vi "Function Template.vi"(8 "Error In":errorcluster, 11 "Data In":T2) -> (0 "Error Out":errorcluster, 3 "Data Out":T2)   [LabVIEW 2019]
doc: "Description of VI"
uses:
  Controls/Data.ctl
  <vilib>/Utility/error.llb/DialogType.ctl
  <vilib>/Utility/miscctls.llb/LVPointTypeDef.ctl
panel:
  out "Control Tab":T1(tab)
  out "Console Out":string
  out "Error Message":string
  out "VI-filename":string
  out "Revision Number":u32
  out "VI Description":string
  out "Callers' Names":string[](array[string])
  out "Code Size":u32
  out "VI Type":T3(ring)
  out "Project name":string
  out "Project filepath":path
  out "VI filepath":path
  out "Project Description":string
  out "VI-Name":string
  # "Common Errors:"
  # "0:"
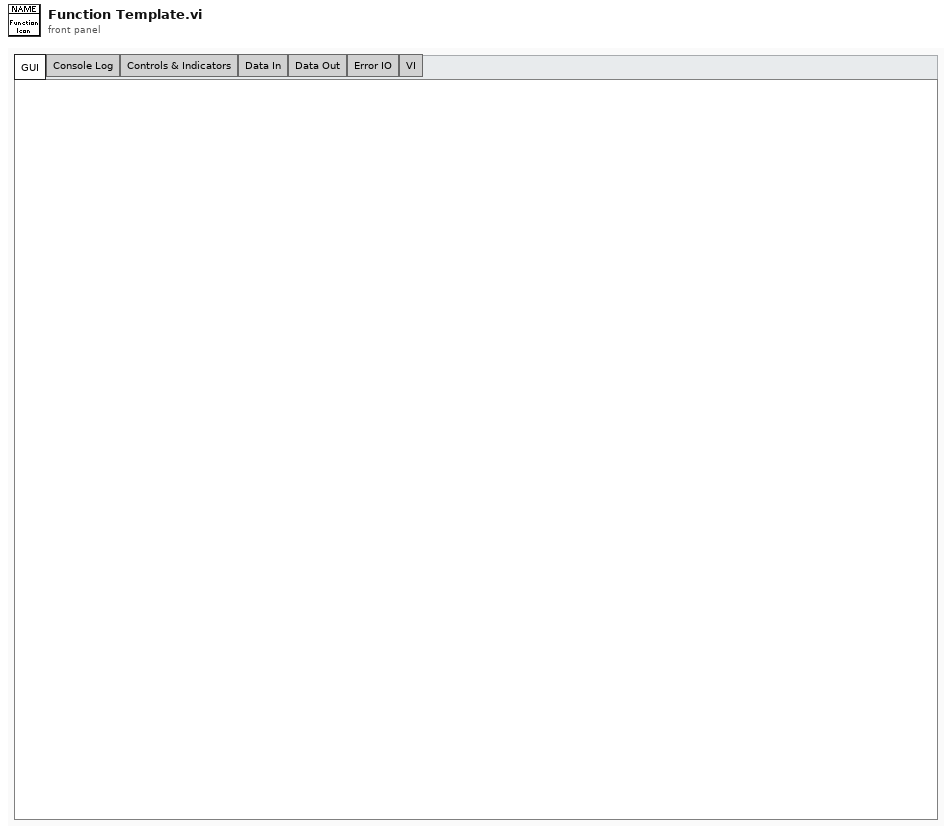
[diagram p1: front panel]
types:
  T1 = enum32{"GUI", "Console Log", "Controls & Indicators", "Data In", "Data Out", "Error IO", "VI"}
  T2 = typedef "Data.ctl" = cluster{"Console log":string}
  T3 = enum32{"invalid VI type", "Standard VI", "Control VI", "Global VI", "Polymorphic VI", "Configuration VI", "SubSystem", "Facade VI", "Method VI", "Statechart Diagram VI"}
  T4 = typedef "LVPointTypeDef.ctl" = cluster{"Horizontal":i16, "Vertical":i16}
  T5 = typedef "DialogType.ctl" = u16
  T6 = typedef "LVRectTypeDef.ctl" = cluster{"Left":i16, "Top":i16, "Right":i16, "Bottom":i16}
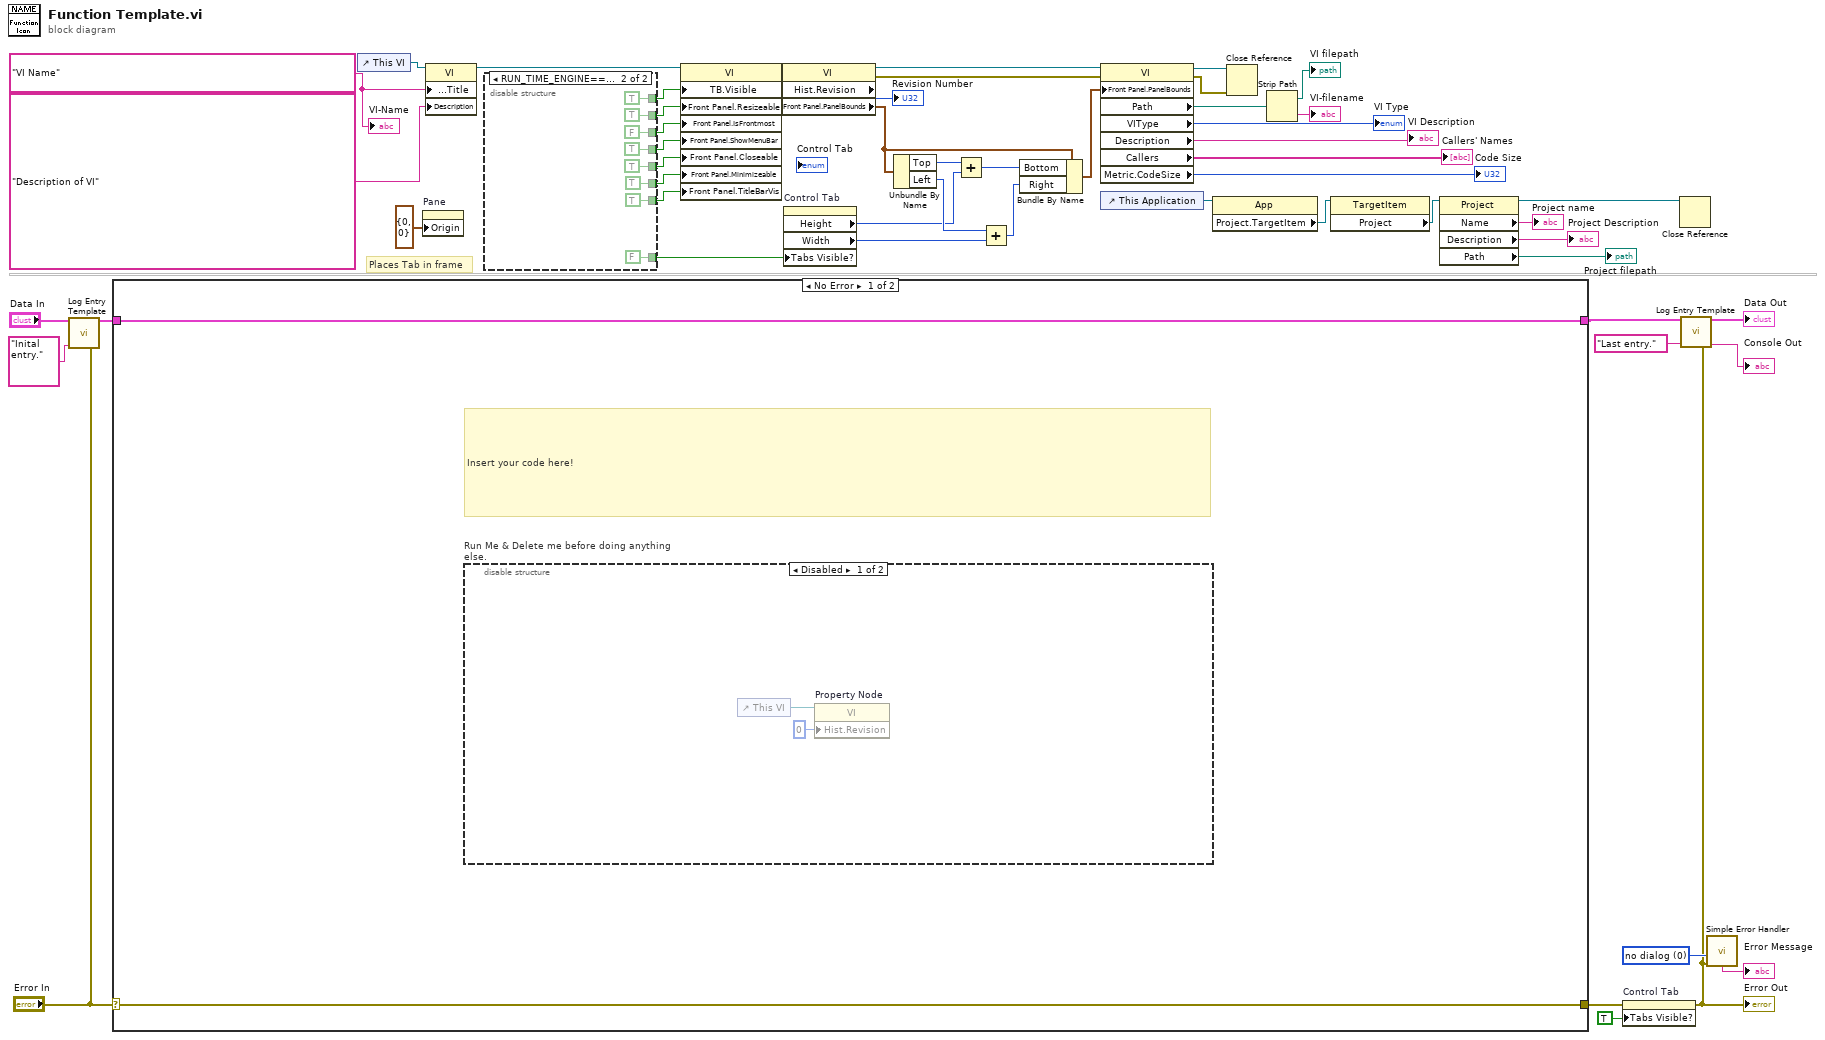
[diagram p0: block diagram]
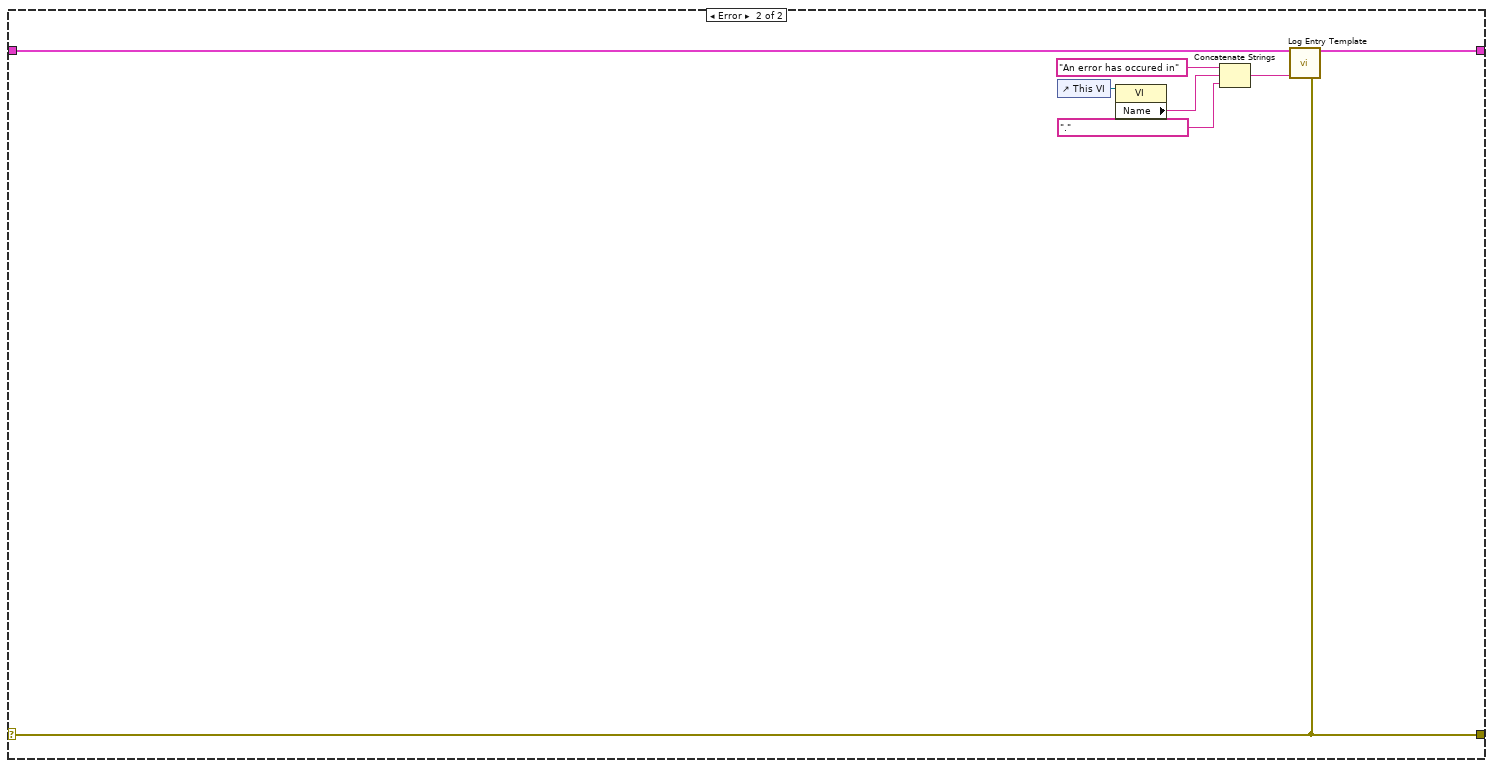
[diagram p3: hidden frame]
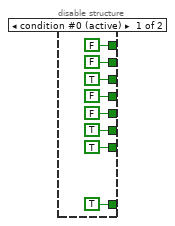
[diagram p4: hidden frame]
diagram:
  w24 = "VI Name"
  w52 = T5 0 items=["no dialog", "OK message", "continue or stop message", "OK message + warnings", "continue/stop + warnings"] ("type of dialog (OK msg:1)")
  # "Places Tab in frame"
  n1 = call "Log Entry Template.vi"("Data In"="Data In", "Console Entry"="Inital entry.", "Error In"="Error In") -> ("Data Out"=w4:T2)  [unwired: 11 in, 1 out]
  n2 = case shown="No Error" "Error In" {
    selector: "Error In" -> [w56 w65]
    tunnel: w4 -> [w57 w66]
    tunnel: [w57 w67] -> w3
    tunnel: [w56 w65] -> w1
    frame No Error {
      # "Insert your code here!"
      n3 = disable-structure "Run Me & Delete me before doing anything else." shown="Disabled" {
        frame Disabled {
          n4 = control-ref of="This VI"() -> (w59:refnum<vi>)
          n5 = property on="Property Node" class="VI"(reference=w59, "Hist.Revision"=u32 0 ("History:Revision Number")) -> ()  [unwired: 1 in, 2 out]
        }
        frame Enabled {
        }
      }
    }
    frame Error {
      n6 = control-ref of="This VI"() -> (w63:refnum<vi>)
      n7 = property class="VI"(reference=w63) -> ("Name"=w62:string)  [unwired: 1 in, 2 out]
      n8 = Concatenate Strings("An error has occured in" ("Console Entry"), w62, "." ("string")) -> (w60:string)
      n9 = call "Log Entry Template.vi"("Data In"=w66, "Console Entry"=w60, "Error In"=w65) -> ("Data Out"=w67:T2)  [unwired: 11 in, 1 out]
    }
  }
  n10 = control-ref of="This VI"() -> (w36:refnum<vi>)
  n11 = property on="Pane" class="Pane"("Origin"=T4 {"Horizontal"=0, "Vertical"=0}) -> ()  [unwired: 2 in, 2 out]
  n12 = property class="VI"(reference=w36, "Front Panel.Title"=w24, "Description"="Description of VI") -> (reference out=w26:refnum<vi>)  [unwired: 1 in, 1 out]
  n13 = disable-structure "Exe vs Sim" shown="RUN_TIME_ENGINE==True" {
    disable-tunnel: [FALSE ("Tool Bar:Visible") TRUE ("Tool Bar:Visible")] -> w35
    disable-tunnel: [FALSE ("Front Panel Window:Resizable") TRUE ("Front Panel Window:Resizable")] -> w34
    disable-tunnel: [TRUE ("Front Panel Window:Is Frontmost") FALSE ("Front Panel Window:Is Frontmost")] -> w33
    disable-tunnel: [FALSE ("Front Panel Window:Show Menu Bar") TRUE ("Front Panel Window:Show Menu Bar")] -> w32
    disable-tunnel: [FALSE ("Front Panel Window:Closeable") TRUE ("Front Panel Window:Closeable")] -> w31
    disable-tunnel: [TRUE ("Front Panel Window:Title Bar Visible") TRUE ("Front Panel Window:Title Bar Visible")] -> w30
    disable-tunnel: [TRUE ("Front Panel Window:Minimizable") TRUE ("Front Panel Window:Minimizable")] -> w29
    disable-tunnel: [TRUE FALSE] -> w25
    frame condition #0 (active) {
    }
    frame condition #1 {
    }
  }
  n14 = property class="VI"(reference=w26, "TB.Visible"=w35, "Front Panel.Resizeable"=w34, "Front Panel.IsFrontmost"=w33, "Front Panel.ShowMenuBar"=w32, "Front Panel.Closeable"=w31, "Front Panel.Minimizeable"=w29, "Front Panel.TitleBarVis"=w30) -> (reference out=w28:refnum<vi>, error out=w27:errorcluster)  [unwired: 1 in]
  n15 = property class="VI"(reference=w28, error in=w27) -> (reference out=w42:refnum<vi>, error out=w38:errorcluster, "Hist.Revision"=→"Revision Number":u32, "Front Panel.PanelBounds"=w43:T6)
  n16 = property on="Control Tab" class="TabCtl (strict)"("Tabs Visible?"=w25) -> ("Height"=w45:u32, "Width"=w49:u32)  [unwired: 2 in, 2 out]
  n17 = Unbundle By Name(w43) -> ("Top"=w44:i16, "Left"=w48:i16)
  n18 = Add(x=w44, y=w45) -> (x+y=w46:u32)
  n19 = Add(x=w48, y=w49) -> (x+y=w47:u32)
  n20 = Bundle By Name(cluster=w43, "Bottom"=w46, "Right"=w47) -> (w41:T6)
  n21 = property on="Window size" class="VI"(reference=w42, error in=w38, "Front Panel.PanelBounds"=w41) -> (reference out=w50:refnum<vi>, error out=w39:errorcluster, "Path"=w23:path, "VIType"=→"VI Type":T3, "Description"=→"VI Description":string, "Callers"=→"Callers' Names":string[], "Metric.CodeSize"=→"Code Size":u32)
  n22 = control-ref of="This Application"() -> (w13:refnum<vi>)
  n23 = property class="App"(reference=w13) -> ("Project.TargetItem"=w18:refnum<vi>)  [unwired: 1 in, 2 out]
  n24 = Close Reference(reference=w50, error in (no error)=w39) -> ()  [unwired: 1 out]
  n25 = Strip Path(path=w23) -> (stripped path=→"VI filepath":path, name=→"VI-filename":string)
  n26 = property class="TargetItem"(reference=w18) -> ("Project"=w17:refnum<vi>)  [unwired: 1 in, 2 out]
  n27 = property class="Project"(reference=w17) -> (reference out=w11:refnum<vi>, "Name"=→"Project name":string, "Description"=→"Project Description":string, "Path"=→"Project filepath":path)  [unwired: 1 in, 1 out]
  n28 = property on="Control Tab" class="TabCtl (strict)"(error in=w1, "Tabs Visible?"=TRUE) -> (error out=w5:errorcluster)  [unwired: 1 in, 1 out]
  "Error Out" <- w5
  n29 = Close Reference(reference=w11) -> ()  [unwired: 1 in, 1 out]
  n30 = call "Log Entry Template.vi"("Data In"=w3, "Console Entry"="Last entry.", "Error In"=w5) -> ("Data Out"=→"Data Out":T2, "Console log out"=→"Console Out":string)  [unwired: 11 in]
  n31 = call <vilib>:"Simple Error Handler.vi"("type of dialog (OK msg:1)"=w52, "error in (no error)"=w5) -> ("message"=→"Error Message":string)  [unwired: 3 in, 4 out]
  "VI-Name" <- w24
